vi "Timestamps with Start and Stop Command.vi"(7 "base name for channel aliases":string, 8 "error in":errorcluster, 11 "Loopback in":refnum<class "Loopback.lvclass">) -> (0 "error out":errorcluster, 3 "Loopback out":refnum<class "Loopback.lvclass">)   [LabVIEW 2020, in "Loopback.lvclass"]
uses:
  Loopback.lvclass
  <vilib>/NI VeriStand/Execution/Workspace/NI_VS Workspace ExecutionAPI.lvlib
  <vilib>/NI VeriStand/Execution/Workspace/NI VeriStand - Get Multiple Channel Values.vi
  <vilib>/NI VeriStand/Execution/Workspace/NI VeriStand - Get Single Channel Value.vi
  2518613e-1aa0-4c19-ab93-1fd17e2112ff.vi
  <vilib>/NI VeriStand/Execution/Workspace/NI VeriStand - Set Single Channel Value.vi
  c9951261-b4e7-445f-95ae-1924f02875ce.vi
  d018f213-e546-4c43-981e-280bd99d7f58.vi
  4066b549-521b-42b3-9963-63becf34a3c7.vi
  b48528fb-317c-4840-992d-cf61b4b6420f.vi
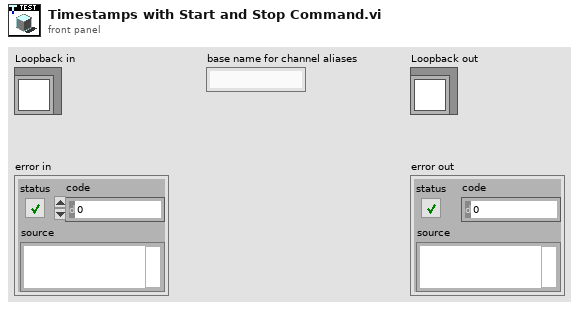
[diagram p1: front panel]
types:
  T1 = typedef "NI_VS Workspace ExecutionAPI.lvlib/WorkspaceAPI.ctl" = refnum<k24>
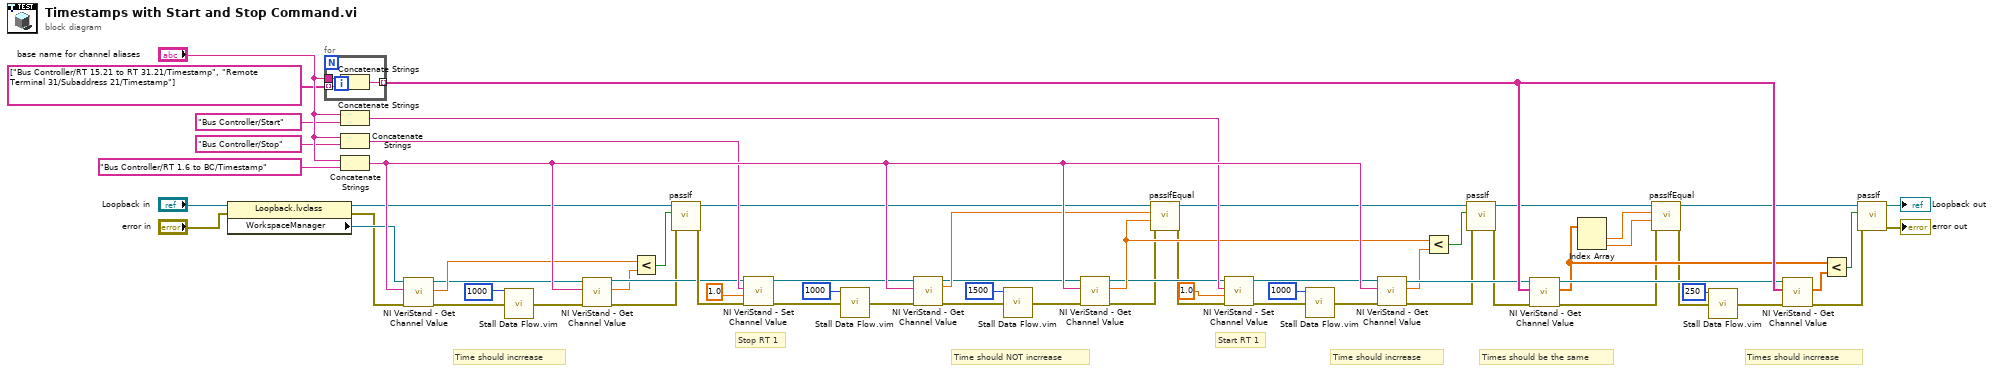
[diagram p0: block diagram]
diagram:
  # "Time should incrrease"
  # "Start RT 1"
  # "Time should NOT incrrease"
  # "Stop RT 1"
  # "Times should incrrease"
  # "Times should be the same"
  # "Time should incrrease"
  n1 = property class="Loopback.lvclass"(reference="Loopback in", error in="error in") -> (reference out=w1:refnum<class "Loopback.lvclass">, error out=w2:errorcluster, "WorkspaceManager"=w3:T1)
  n2 = for {
    tunnel: string[] ["Bus Controller/RT 15.21 to RT 31.21/Timestamp", "Remote Terminal 31/Subaddress 21/Timestamp"] ("Channels") -> [w68] mode=indexing
    tunnel: "base name for channel aliases" -> [w67]
    tunnel: [w66] -> w61 mode=indexing
    n3 = Concatenate Strings(w67, w68) -> (w66:string)
  }
  n4 = Concatenate Strings("base name for channel aliases", "Bus Controller/Start" ("Channel")) -> (w56:string)
  n5 = Concatenate Strings("base name for channel aliases", "Bus Controller/Stop" ("Channel")) -> (w58:string)
  n6 = Concatenate Strings("base name for channel aliases", "Bus Controller/RT 1.6 to BC/Timestamp") -> (w62:string)
  n7 = call-poly <vilib>:"NI VeriStand - Get Channel Value.vi"("error in (no error)"=w2, "Channel"=w62, "WorkspaceManager in"=w3) -> ("error out"=w8:errorcluster, "Value"=w12:dbl, "WorkspaceManager out"=w6:T1)  [unwired: 6 in]
  n8 = call "Stall Data Flow.vim"("value in"=w8, "milliseconds to wait"=u32 1000) -> ("value out"=w7:errorcluster)  [unwired: 1 out]
  n9 = call-poly <vilib>:"NI VeriStand - Get Channel Value.vi"("error in (no error)"=w7, "Channel"=w62, "WorkspaceManager in"=w6) -> ("error out"=w10:errorcluster, "Value"=w13:dbl, "WorkspaceManager out"=w29:T1)  [unwired: 6 in]
  n10 = Less?(x=w12, y=w13) -> (x < y?=w14:bool)
  n11 = call-dynamic "passIf.vi"("error in (no error)"=w10, "pass"=w14, "TestCase in"=w1) -> ("error out"=w30:errorcluster, "TestCase out"=w37:refnum<class "Loopback.lvclass">)  [unwired: 7 in]
  n12 = call-poly <vilib>:"NI VeriStand - Set Channel Value.vi"("error in (no error)"=w30, "Value"=1.0, "Channel"=w58, "WorkspaceManager in"=w29) -> ("error out"=w27:errorcluster, "WorkspaceManager out"=w33:T1)  [unwired: 6 in]
  n13 = call "Stall Data Flow.vim"("value in"=w27, "milliseconds to wait"=u32 1000) -> ("value out"=w34:errorcluster)  [unwired: 1 out]
  n14 = call-poly <vilib>:"NI VeriStand - Get Channel Value.vi"("error in (no error)"=w34, "Channel"=w62, "WorkspaceManager in"=w33) -> ("error out"=w32:errorcluster, "Value"=w38:dbl, "WorkspaceManager out"=w35:T1)  [unwired: 6 in]
  n15 = call "Stall Data Flow.vim"("value in"=w32, "milliseconds to wait"=u32 1500) -> ("value out"=w36:errorcluster)  [unwired: 1 out]
  n16 = call-poly <vilib>:"NI VeriStand - Get Channel Value.vi"("error in (no error)"=w36, "Channel"=w62, "WorkspaceManager in"=w35) -> ("error out"=w39:errorcluster, "Value"=w49:dbl, "WorkspaceManager out"=w45:T1)  [unwired: 6 in]
  n17 = call-dynamic "passIfEqual.vi"("error in (no error)"=w39, "y"=w49, "x"=w38, "TestCase in"=w37) -> ("error out"=w44:errorcluster, "TestCase out"=w50:refnum<class "Loopback.lvclass">)  [unwired: 6 in]
  n18 = call-poly <vilib>:"NI VeriStand - Set Channel Value.vi"("error in (no error)"=w44, "Value"=1.0, "Channel"=w56, "WorkspaceManager in"=w45) -> ("error out"=w42:errorcluster, "WorkspaceManager out"=w40:T1)  [unwired: 6 in]
  n19 = call "Stall Data Flow.vim"("value in"=w42, "milliseconds to wait"=u32 1000) -> ("value out"=w46:errorcluster)  [unwired: 1 out]
  n20 = call-poly <vilib>:"NI VeriStand - Get Channel Value.vi"("error in (no error)"=w46, "Channel"=w62, "WorkspaceManager in"=w40) -> ("error out"=w51:errorcluster, "Value"=w48:dbl, "WorkspaceManager out"=w53:T1)  [unwired: 6 in]
  n21 = Less?(x=w49, y=w48) -> (x < y?=w47:bool)
  n22 = call-dynamic "passIf.vi"("error in (no error)"=w51, "pass"=w47, "TestCase in"=w50) -> ("error out"=w52:errorcluster, "TestCase out"=w54:refnum<class "Loopback.lvclass">)  [unwired: 7 in]
  n23 = call-poly <vilib>:"NI VeriStand - Get Channel Value.vi"("error in (no error)"=w52, "Channels"=w61, "WorkspaceManager in"=w53) -> ("error out"=w11:errorcluster, "Values"=w22:dbl[], "WorkspaceManager out"=w24:T1)  [unwired: 6 in]
  n24 = Index Array(array=w22) -> (element #1=w15:dbl, element #2=w16:dbl)  [unwired: 2 in]
  n25 = call-dynamic "passIfEqual.vi"("error in (no error)"=w11, "y"=w16, "x"=w15, "TestCase in"=w54) -> ("error out"=w17:errorcluster, "TestCase out"=w25:refnum<class "Loopback.lvclass">)  [unwired: 6 in]
  n26 = call "Stall Data Flow.vim"("value in"=w17, "milliseconds to wait"=u32 250) -> ("value out"=w19:errorcluster)  [unwired: 1 out]
  n27 = call-poly <vilib>:"NI VeriStand - Get Channel Value.vi"("error in (no error)"=w19, "Channels"=w61, "WorkspaceManager in"=w24) -> ("error out"=w21:errorcluster, "Values"=w23:dbl[])  [unwired: 6 in, 1 out]
  n28 = Less?(x=w22, y=w23) -> (x < y?=w20:bool)
  n29 = call-dynamic "passIf.vi"("error in (no error)"=w21, "pass"=w20, "TestCase in"=w25) -> ("error out"=→"error out":errorcluster, "TestCase out"=→"Loopback out":refnum<class "Loopback.lvclass">)  [unwired: 7 in]
